vi "ABR-Options Dialog.vi"(0 "Hidden":T3={"AI Samp Rate Hz"=0.0, "AO Samp Rate Hz"=100000.0, "Duration (ms)"=5.0, "Ramp (ms)"=0.5, "Click width (us)"=0.0, "ITI"=enum."Rate", "Save raw"=FALSE}, 2 "Parent VI":refnum<vi>, 5 "Threshold Estimation In":T2) -> (4 "Cluster out":T3={"AI Samp Rate Hz"=0.0, "AO Samp Rate Hz"=100000.0, "Duration (ms)"=5.0, "Ramp (ms)"=0.5, "Click width (us)"=0.0, "ITI"=enum."Rate", "Save raw"=FALSE}, 6 "Threshold Estimation Out":T2, 8 "Canceled?":bool)   [LabVIEW 2020]
uses:
  TypeDefs/ABR-Hidden Params.ctl
  Threshold Estimation VIs/ABR3-Threshold Estimation Parameters.ctl
  epl-vi-lib/Utility VIs/Buttons/KCheckmarkBoolean 2.ctl
panel:
  in  "Save raw data":T1
  out "exit signal":bool
  in  "ITI":enum16{"Rate", "Interval"}(ring) caption="Express intertrial timing as"
  in  "AI Fs":dbl caption="Input sampling rate (Hz)"
  in  "R2 criterion":dbl caption="Adj R2 criterion"
  in  "CC criterion":dbl caption="Corrcoef criterion"
  in  "Thr Tmax":dbl caption="Tmax (ms)"
  in  "Thr Tmin":dbl caption="Tmin (ms)"
  in  "ClickWidth":dbl caption="Click duration (us)"
  in  "ToneRamp":dbl caption="Tone burst ramp length (ms)"
  in  "ToneDur":dbl caption="Tone burst duration (ms)"
  in  "AO Fs":dbl caption="Output sampling rate (Hz)"
  in  "Cancel":bool
  in  "OK":bool
  # "Threshold estimation"
  # "Warning! Unless you're sure you know what you're doing, don't change these parameters"
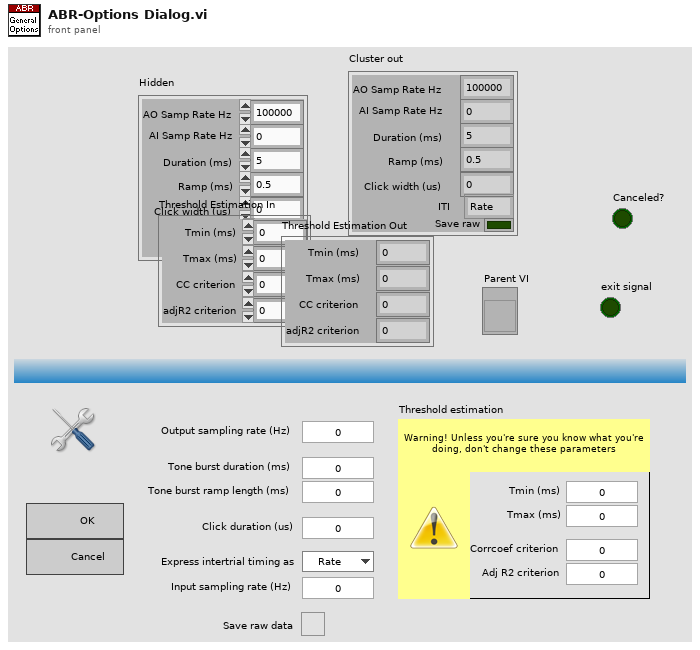
[diagram p1: front panel]
types:
  T1 = typedef "KCheckmarkBoolean 2.ctl" = bool
  T2 = typedef "ABR3-Threshold Estimation Parameters.ctl" = cluster{"Tmin (ms)":dbl, "Tmax (ms)":dbl, "CC criterion":dbl, "adjR2 criterion":dbl}
  T3 = typedef "ABR-Hidden Params.ctl" = cluster{"AI Samp Rate Hz":dbl, "AO Samp Rate Hz":dbl, "Duration (ms)":dbl, "Ramp (ms)":dbl, "Click width (us)":dbl, "ITI":enum16{"Rate", "Interval"}, "Save raw":bool}
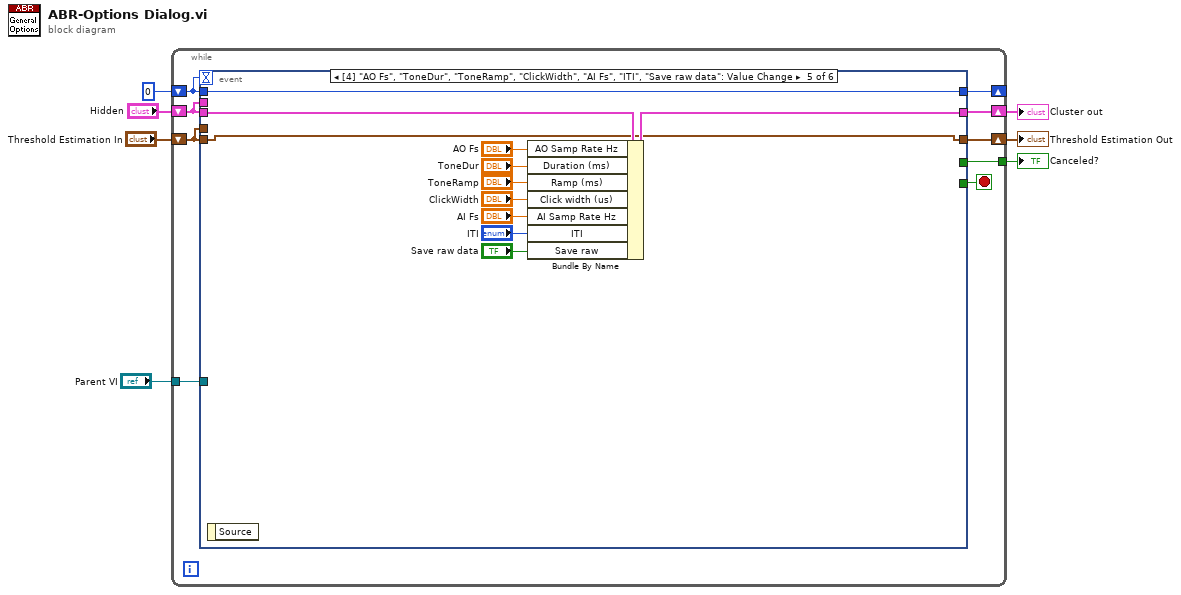
[diagram p0: block diagram]
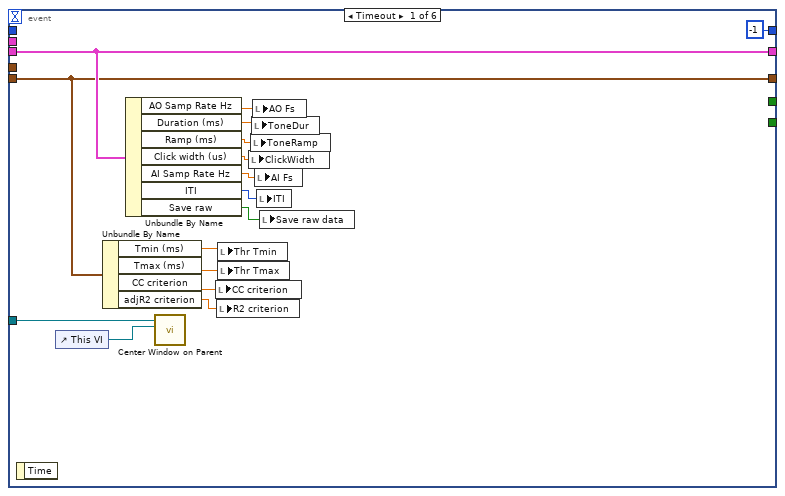
[diagram p2: hidden frame]
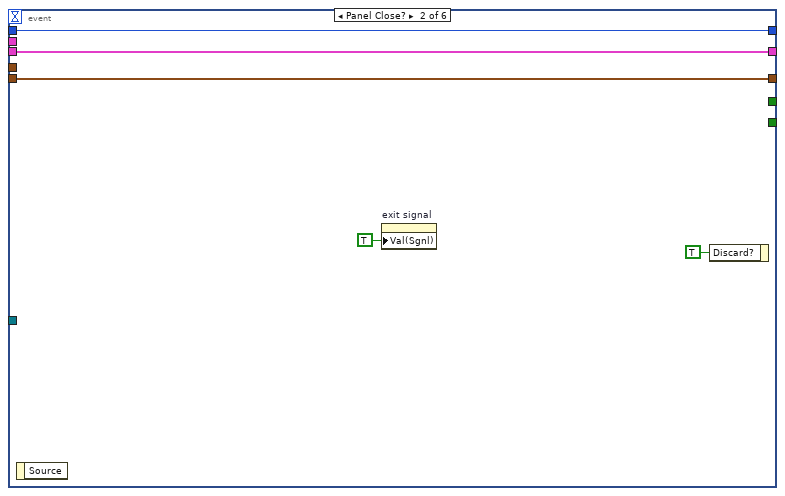
[diagram p3: hidden frame]
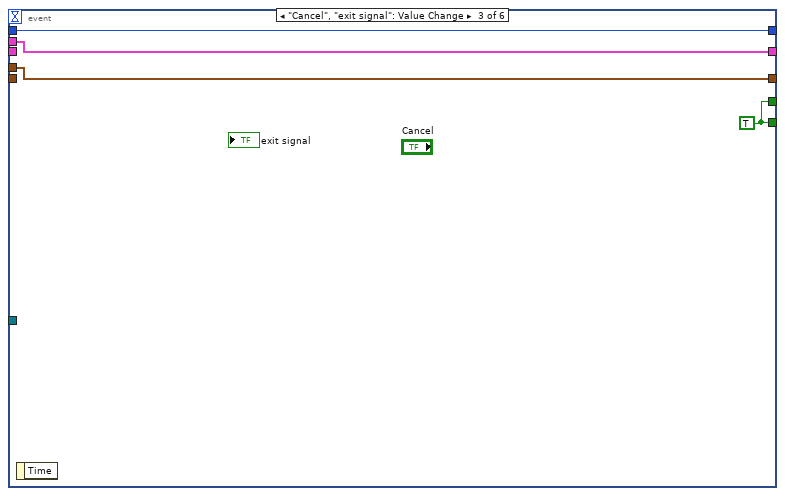
[diagram p4: hidden frame]
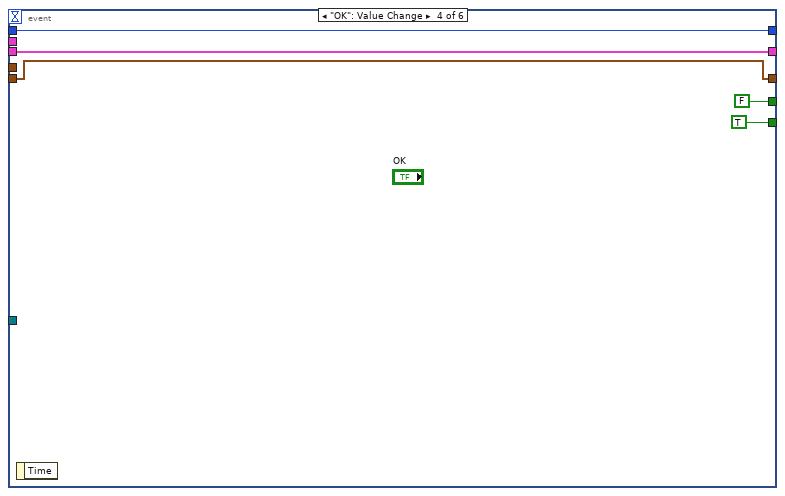
[diagram p5: hidden frame]
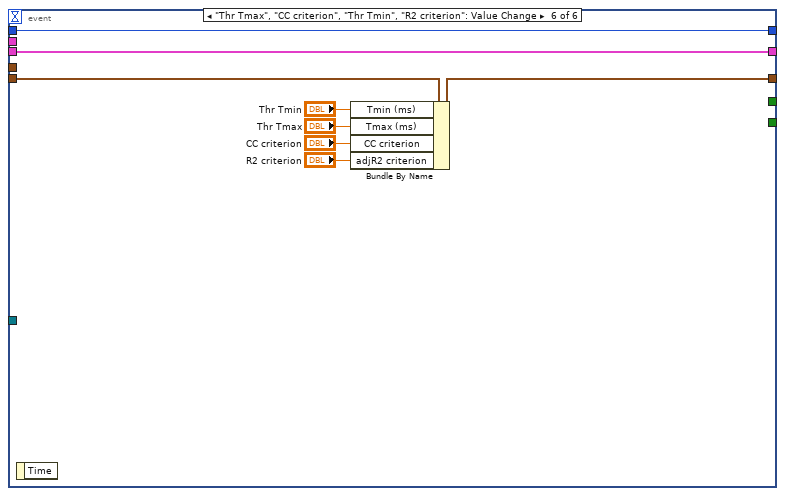
[diagram p6: hidden frame]
diagram:
  n1 = while {
    shift-right: [w16] -> _
    shift-left: 0 -> [w9]
    tunnel: [w13] -> w4
    shift-right: [w15] -> w5
    shift-left: "Hidden" -> [w12]
    shift-right: [w11] -> w2
    shift-left: "Threshold Estimation In" -> [w10]
    tunnel: "Parent VI" -> [w8]
    stop <- w14 stop-if-true
    n2 = event shown="[4] \"AO Fs\", \"ToneDur\", \"ToneRamp\", \"ClickWidth\", \"AI Fs\", \"ITI\", \"Save raw data\": Value Change" {
      selector: _ -> [_ _ _ _ _ _]
      dyn-events: _ -> [_ _ _ _ _ _]
      timeout: w9 -> [_ _ _ _ _ _]
      tunnel: [-1 w37 w38 w42 w50 w61] -> w16
      tunnel: w12 -> [w31 w33 _ w46 w57 w65]
      tunnel: [w31 w33 w40 w46 w56 w65] -> w15
      tunnel: [_ _ w41 TRUE _ _] -> w14
      tunnel: [_ _ w41 FALSE _ _] -> w13
      tunnel: w12 -> [_ _ w40 _ _ _]
      tunnel: w10 -> [w26 w36 _ w43 w51 w59]
      tunnel: [w26 w36 w39 w43 w51 w58] -> w11
      tunnel: w10 -> [_ _ w39 _ _ _]
      tunnel: w9 -> [_ w37 w38 w42 w50 w61]
      tunnel: w8 -> [w22 _ _ _ _ _]
      event Timeout {
        n3 = event-data() -> ()  [unwired: 1 in, 1 out]
        n4 = control-ref of="This VI"() -> (w21:refnum<vi>)
        n5 = Unbundle By Name(w26) -> ("Tmin (ms)"=w25:dbl, "Tmax (ms)"=w24:dbl, "CC criterion"=w23:dbl, "adjR2 criterion"=w20:dbl)
        n6 = Unbundle By Name(w31) -> ("AO Samp Rate Hz"=w30:dbl, "Duration (ms)"=w29:dbl, "Ramp (ms)"=w28:dbl, "Click width (us)"=w27:dbl, "AI Samp Rate Hz"=w19:dbl, "ITI"=w18:enum16{"Rate", "Interval"}, "Save raw"=w17:bool)
        n7 = call "Center Window on Parent.vi"("Parent VI"=w21, "VI in"=w22) -> ()  [unwired: 8 in, 2 out]
        n8 = local write "CC criterion"(w23) -> ()
        n9 = local write "R2 criterion"(w20) -> ()
        n10 = local write "Thr Tmin"(w25) -> ()
        n11 = local write "Thr Tmax"(w24) -> ()
        n12 = local write "ClickWidth"(w27) -> ()
        n13 = local write "ToneRamp"(w28) -> ()
        n14 = local write "ToneDur"(w29) -> ()
        n15 = local write "AO Fs"(w30) -> ()
        n16 = local write "AI Fs"(w19) -> ()
        n17 = local write "ITI"(w18) -> ()
        n18 = local write "Save raw data"(w17) -> ()
      }
      event Panel Close? {
        n19 = event-data() -> ()  [unwired: 1 in, 1 out]
        n20 = property on="exit signal" class="Bool (strict)"("Val(Sgnl)"=TRUE ("Value (Signaling)")) -> ()  [unwired: 2 in, 2 out]
        n21 = event-data("Discard?"=TRUE) -> ()  [unwired: 1 in, 1 out]
      }
      event "Cancel", "exit signal": Value Change {
        w41 = TRUE
        n22 = event-data() -> ()  [unwired: 1 in, 1 out]
      }
      event "OK": Value Change {
        n23 = event-data() -> ()  [unwired: 1 in, 1 out]
      }
      event "AO Fs", "ToneDur", "ToneRamp", "ClickWidth", "AI Fs", "ITI": Value Change {
        n24 = event-data() -> ()  [unwired: 1 in, 1 out]
        n25 = Bundle By Name(cluster=w57, "AO Samp Rate Hz"="AO Fs", "Duration (ms)"="ToneDur", "Ramp (ms)"="ToneRamp", "Click width (us)"="ClickWidth", "AI Samp Rate Hz"="AI Fs", "ITI"="ITI", "Save raw"="Save raw data") -> (w56:T3)
      }
      event "Thr Tmax", "CC criterion", "Thr Tmin", "R2 criterion": Value Change {
        n26 = event-data() -> ()  [unwired: 1 in, 1 out]
        n27 = Bundle By Name(cluster=w59, "Tmin (ms)"="Thr Tmin", "Tmax (ms)"="Thr Tmax", "CC criterion"="CC criterion", "adjR2 criterion"="R2 criterion") -> (w58:T2)
      }
    }
  }
  "Cluster out" <- w5
  "Canceled?" <- w4
  "Threshold Estimation Out" <- w2
